vi "Generador_DAQ_1.vi"() -> ()   [LabVIEW 2015]
uses:
  <vilib>/DAQmx/write.llb/DAQmx Write (Analog 1D DBL 1Chan NSamp).vi
  <vilib>/DAQmx/create/channels.llb/DAQmx Create Channel (AO-Voltage-Basic).vi
  <vilib>/DAQmx/configure/timing.llb/DAQmx Timing (Sample Clock).vi
  <vilib>/DAQmx/miscellaneous.llb/DAQmx Fill In Error Info.vi
panel:
  out "Waveform Graph":dbl[](graph)
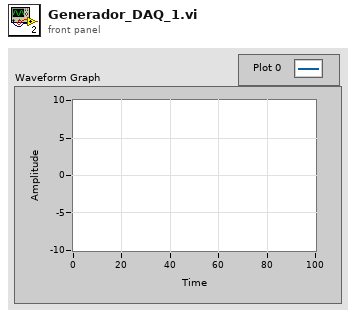
[diagram p1: front panel]
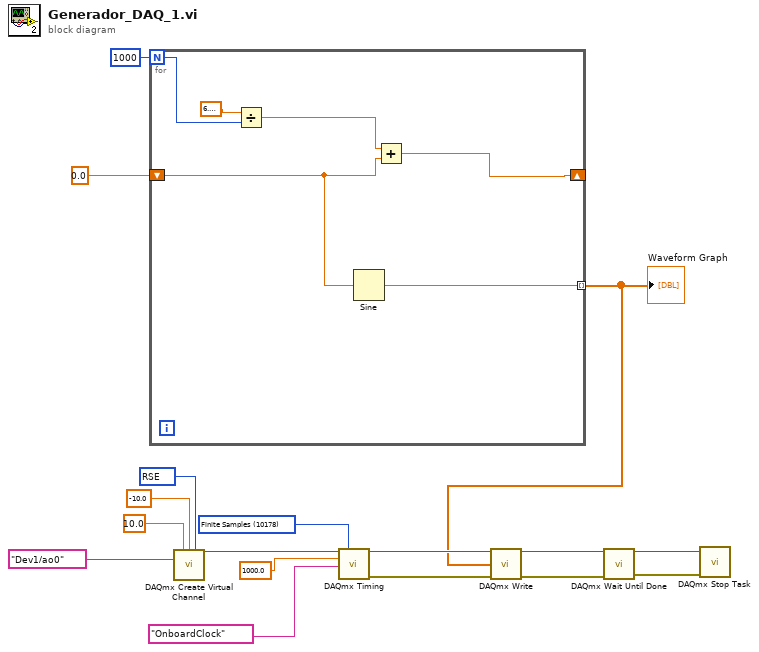
[diagram p0: block diagram]
diagram:
  w10 = 10178 items=["Finite Samples"=10178, "Continuous Samples"=10123, "Hardware Timed Single Point"=12522] ("sample mode")
  w15 = 10083 items=["Default"=-1, "RSE"=10083, "Differential"=10106, "Pseudodifferential"=12529] ("output terminal configuration")
  n1 = for {
    N: 1000 -> [w22]
    shift-right: [w20] -> _
    shift-left: 0.0 -> [w19]
    tunnel: [w18] -> w5 mode=indexing
    n2 = Divide(x=6.283185307179586, y=w22) -> (x/y=w21:dbl)
    n3 = Sine(x=w19) -> (sin(x)=w18:dbl)
    n4 = Add(x=w21, y=w19) -> (x+y=w20:dbl)
  }
  "Waveform Graph" <- w5
  n5 = call-poly <vilib>:"DAQmx Create Virtual Channel.vi"("maximum value"=10.0, "minimum value"=-10.0, "output terminal configuration"=w15, "physical channels"=tag "Dev1/ao0") -> ("task out"=w12:refnum<k21>)  [unwired: 10 in, 1 out]
  n6 = call-poly <vilib>:"DAQmx Timing.vi"("task/channels in"=w12, "sample mode"=w10, "rate"=1000.0, "source"=tag "OnboardClock") -> ("task out"=w7:refnum<k21>, "error out"=w6:errorcluster)  [unwired: 10 in]
  n7 = call-poly <vilib>:"DAQmx Write.vi"("task/channels in"=w7, "data"=w5, "error in"=w6) -> ("task out"=w4:refnum<k21>, "error out"=w3:errorcluster)  [unwired: 10 in, 1 out]
  n8 = call <vilib>:"DAQmx Wait Until Done.vi"("task/channels in"=w4, "error in"=w3) -> ("task out"=w2:refnum<k21>, "error out"=w1:errorcluster)  [unwired: 12 in]
  n9 = call <vilib>:"DAQmx Stop Task.vi"("task/channels in"=w2, "error in"=w1) -> ()  [unwired: 12 in, 2 out]
